vi "Stacked Secuence.vi"() -> ()   [LabVIEW 2020]
panel:
  out "Tank 5":dbl(slide) scale=0.0..100.0
  out "Tank 4":dbl(slide) scale=0.0..100.0
  out "Tank 3":dbl(slide) scale=0.0..100.0
  out "Tank 2":dbl(slide) scale=0.0..100.0
  out "Tank":dbl(slide) scale=0.0..100.0
  # "STACKED SECUENCE"
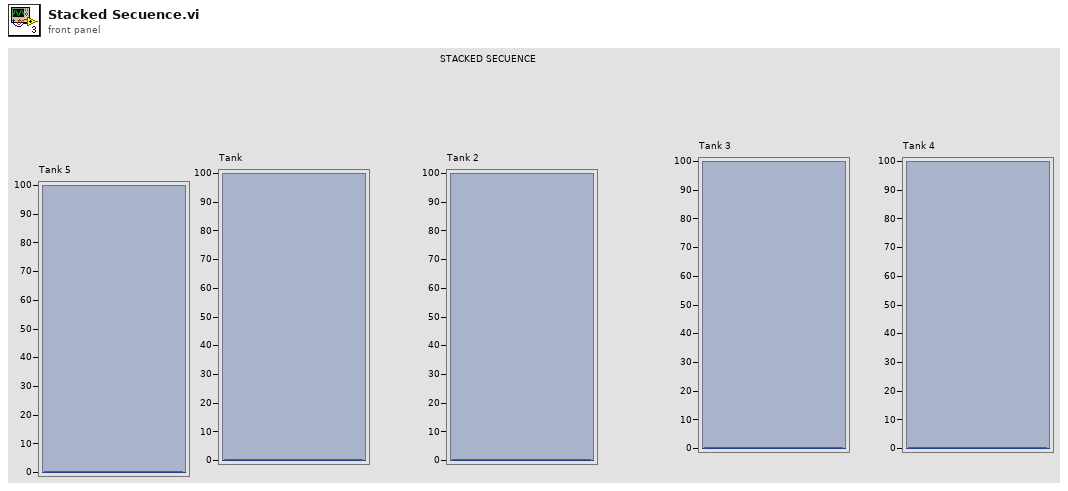
[diagram p1: front panel]
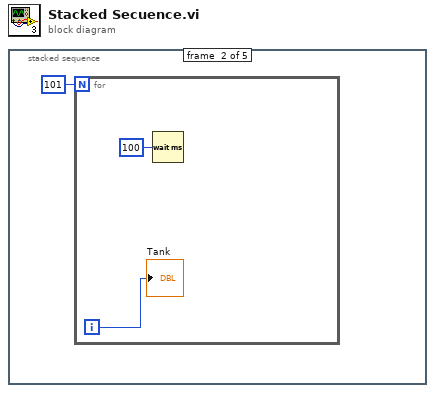
[diagram p0: block diagram]
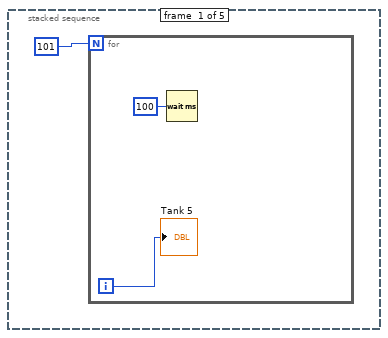
[diagram p2: hidden frame]
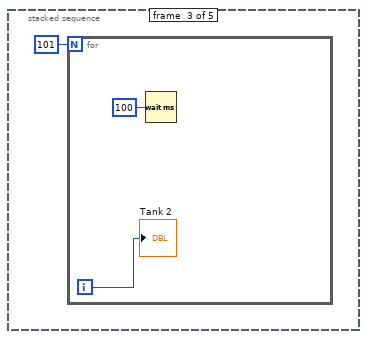
[diagram p3: hidden frame]
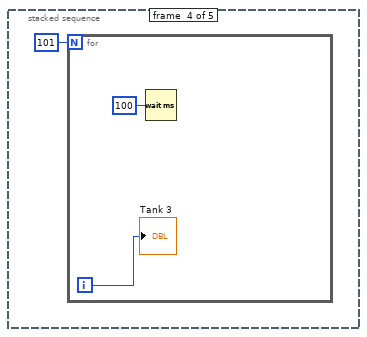
[diagram p4: hidden frame]
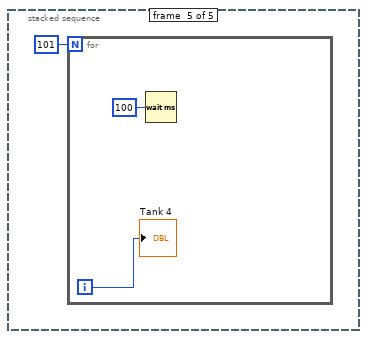
[diagram p5: hidden frame]
diagram:
  n1 = stacked-sequence {
    frame #0 {
      n2 = for {
        N: 101 -> [_]
        i -> [w3]
        n3 = Wait (ms)(milliseconds to wait=u32 100) -> ()  [unwired: 1 out]
        "Tank 5" <- w3
      }
    }
    frame #1 {
      n4 = for {
        N: 101 -> [_]
        i -> [w6]
        n5 = Wait (ms)(milliseconds to wait=u32 100) -> ()  [unwired: 1 out]
        "Tank" <- w6
      }
    }
    frame #2 {
      n6 = for {
        N: 101 -> [_]
        i -> [w9]
        n7 = Wait (ms)(milliseconds to wait=u32 100) -> ()  [unwired: 1 out]
        "Tank 2" <- w9
      }
    }
    frame #3 {
      n8 = for {
        N: 101 -> [_]
        i -> [w12]
        n9 = Wait (ms)(milliseconds to wait=u32 100) -> ()  [unwired: 1 out]
        "Tank 3" <- w12
      }
    }
    frame #4 {
      n10 = for {
        N: 101 -> [_]
        i -> [w15]
        n11 = Wait (ms)(milliseconds to wait=u32 100) -> ()  [unwired: 1 out]
        "Tank 4" <- w15
      }
    }
  }
